vi "Get_Information_Operator_Blinking.vi"(8 "error in (no error)":errorcluster caption="entrée d'erreur (pas d'erreur)", 11 "Class Popup Operator_Validation (Default) en entrée":refnum<class "Class Popup Operator_Validation (Virtual).lvclass">) -> (0 "error out":errorcluster caption="sortie d'erreur", 2 "Information_Operator_Blinking":bool, 3 "Class Popup Operator_Validation (Default) en sortie":refnum<class "Class Popup Operator_Validation (Virtual).lvclass">)   [LabVIEW 2020, in "Library Instrument & Equipement.lvlib" / "Library Popup.lvlib" / "Class Popup Operator_Validation (Virtual).lvclass"]
uses:
  Class Popup Operator_Validation (Virtual).lvclass
  Class Popup Operator_Validation (Virtual).lvclass/Class Popup Operator_Validation (Virtual).ctl
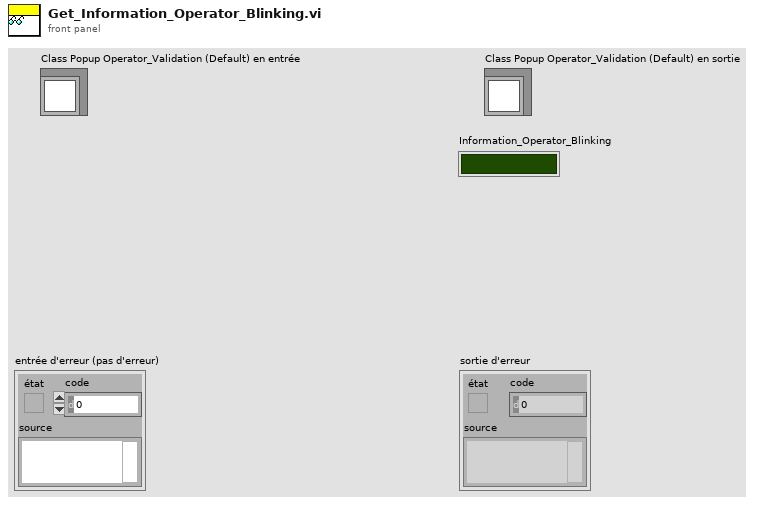
[diagram p1: front panel]
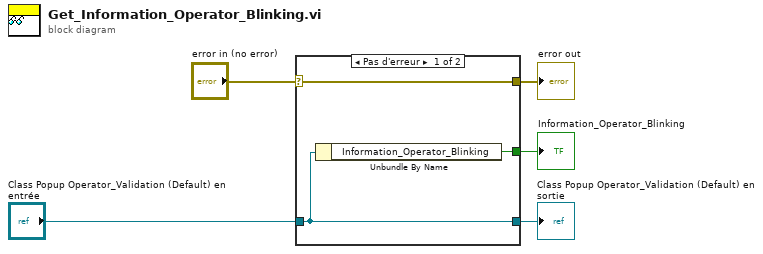
[diagram p0: block diagram]
diagram:
  n1 = case shown="Pas d'erreur" "error in (no error)" {
    selector: "error in (no error)" -> [w8 w9]
    tunnel: [w8 w9] -> w4
    tunnel: [w7 w10] -> w1
    tunnel: "Class Popup Operator_Validation (Default) en entrée" -> [w7 w10]
    tunnel: [w6 _] -> w3
    frame No Error {
      n2 = Unbundle By Name(w7) -> ("Information_Operator_Blinking"=w6:bool)
    }
    frame Error {
    }
  }
  "error out" <- w4
  "Information_Operator_Blinking" <- w3
  "Class Popup Operator_Validation (Default) en sortie" <- w1
